vi "ep_Generate Part Load Efficiency.vi"(8 "error in (no error)":errorcluster, 11 "efficiency values in [%]":dbl[](array[numeric])) -> (0 "error out":errorcluster, 3 "efficiency values out [%]":dbl[](array[numeric]))   [LabVIEW 2014, in "NI_EP_Motor Monitoring.lvlib"]
uses:
  <vilib>/addons/Electrical Power/Motor Monitoring/NI_EP_Motor Monitoring.lvlib
  <vilib>/gmath/NI_Gmath.lvlib
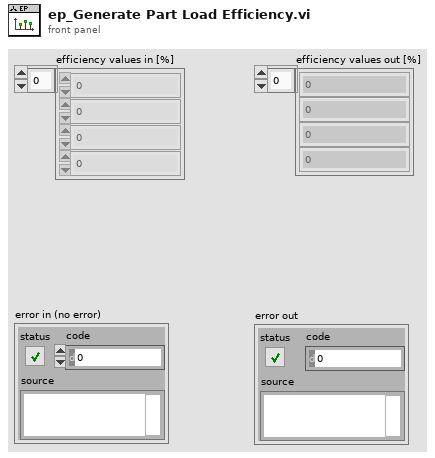
[diagram p1: front panel]
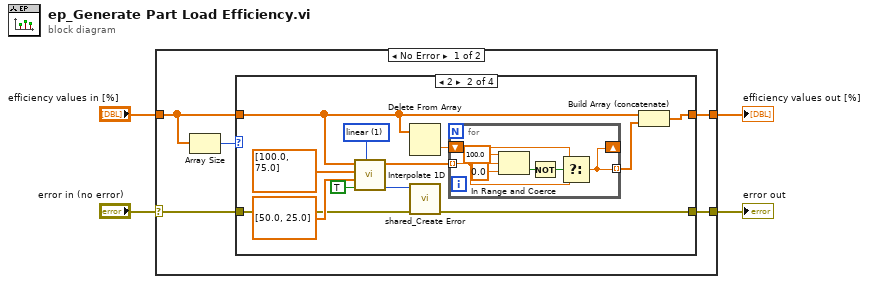
[diagram p0: block diagram]
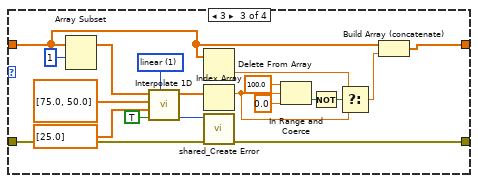
[diagram p3: hidden frame]
diagram:
  n1 = case shown="No Error" "error in (no error)" {
    selector: "error in (no error)" -> [w6 w52]
    tunnel: [w5 w52] -> w3
    tunnel: "efficiency values in [%]" -> [w8 _]
    tunnel: [w7 _] -> w1
    frame No Error {
      n2 = Array Size(array=w8) -> (size(s)=w9:i32)
      n3 = case shown="2" w9 {
        tunnel: w8 -> [w11 w14 w38 w51]
        tunnel: [w11 w20 w46 w51] -> w7
        tunnel: w6 -> [w10 w17 w43 w50]
        tunnel: [w10 w18 w44 w50] -> w5
        frame 1, Default {
        }
        frame 2 {
          w15 = 1 items=["nearest", "linear", "spline", "cubic Hermite", "Lagrange"] ("method")
          n4 = call <vilib>:"Interpolate 1D.vi"("method"=w15, "X is monotonic"=TRUE, "xi"=dbl[] [50.0, 25.0], "X"=dbl[] [100.0, 75.0], "Y"=w14) -> ("error"=w19:i32, "yi"=w16:dbl[])  [unwired: 4 in, 1 out]
          n5 = Delete From Array(array=w14) -> (deleted portion=w13:dbl)  [unwired: 2 in, 1 out]
          n6 = call <vilib>:"shared_Create Error.vi"("error in (no error)"=w17, "error code (0)"=w19) -> ("error out"=w18:errorcluster)  [unwired: 9 in]
          n7 = for {
            tunnel: w16 -> [w27] mode=indexing
            shift-right: [w28] -> _
            shift-left: w13 -> [w29]
            tunnel: [w28] -> w12 mode=indexing
            n8 = In Range and Coerce(upper limit=100.0, x=w27, lower limit=0.0) -> (In Range?=w30:bool)  [unwired: 1 out]
            n9 = Not(x=w30) -> (.not. x?=w24:bool)
            n10 = Select(t=w29, s=w24, f=w27) -> (s? t:f=w28:dbl)
          }
          n11 = Build Array (concatenate)(w14, w12) -> (w20:dbl[])
        }
        frame 3 {
          w39 = 1 items=["nearest", "linear", "spline", "cubic Hermite", "Lagrange"] ("method")
          n12 = Array Subset(array=w38, index=1) -> (w42:dbl[])  [unwired: 1 in]
          n13 = call <vilib>:"Interpolate 1D.vi"("method"=w39, "X is monotonic"=TRUE, "xi"=dbl[] [25.0], "X"=dbl[] [75.0, 50.0], "Y"=w42) -> ("error"=w45:i32, "yi"=w40:dbl[])  [unwired: 4 in, 1 out]
          n14 = Delete From Array(array=w38) -> (deleted portion=w35:dbl)  [unwired: 2 in, 1 out]
          n15 = Index Array(array=w40) -> (element=w34:dbl)  [unwired: 1 in]
          n16 = call <vilib>:"shared_Create Error.vi"("error in (no error)"=w43, "error code (0)"=w45) -> ("error out"=w44:errorcluster)  [unwired: 9 in]
          n17 = In Range and Coerce(upper limit=100.0, x=w34, lower limit=0.0) -> (In Range?=w37:bool)  [unwired: 1 out]
          n18 = Not(x=w37) -> (.not. x?=w31:bool)
          n19 = Select(t=w35, s=w31, f=w34) -> (s? t:f=w36:dbl)
          n20 = Build Array (concatenate)(w38, w36) -> (w46:dbl[])
        }
        frame 4 {
        }
      }
    }
    frame Error {
    }
  }
  "error out" <- w3
  "efficiency values out [%]" <- w1
